vi "4461 Sim - Noise.vi"(4 "Noise Cluster":T1={"1/f vs. Uniform "=1.0, "DC Drift Fraction"=0.0, "DC Drift Freq"=0.19999999999999996, "DC Offset"=0.0, "60Hz Amplitude"=0.005, "Gauss/Unif %"=0.5, "Sig Amp"=1.0, "Noise Amp"=0.005} {"Noise Amp" format="%.1p"; "Sig Amp" format="%.2p"; "Gauss/Unif %" min=0.0 max=1.0 step=0.05 format="%.2f"; "60Hz Amplitude" min=0.0 max=10.0 step=0.05 format="%.2p"; "DC Offset" min=-1.0 max=1.0 step=0.01 format="%.2f"; "DC Drift Freq" min=0.0 max=5.0 step=0.05 format="%.2f"; "DC Drift Fraction" format="%.2f"; "1/f vs. Uniform" min=0.0 max=50.0 step=0.5 format="%.1p"}, 5 "data":waveform(dbl)[](array[waveform]), 6 "sampling info":cluster{"Fs":dbl, "#s":dbl}={"Fs"=204800.0, "#s"=20480.0}) -> (0 "Data":waveform(dbl)[](array[waveform]))   [LabVIEW 2016]
uses:
  <vilib>/Analysis/2dsp.llb/Real FFT.vi
  <vilib>/Analysis/2dsp.llb/Inverse Real FFT.vi
  <vilib>/Analysis/2dsp.llb/Decimate (single shot).vi
  <vilib>/Analysis/2dsp.llb/Decimate (single shot, DBL).vi
  <vilib>/Analysis/3filter.llb/Butterworth Filter (DBL).vi
  <vilib>/Utility/error.llb/Error Cluster From Error Code.vi
  <vilib>/measure/NI_MABase.lvlib
  <vilib>/Analysis/NI_AALPro.lvlib
  <vilib>/Analysis/NI_AALBase.lvlib
panel:
  out "Waveform Graph 2":waveform(dbl)[](graph)
  out "Waveform Graph":waveform(dbl)[](graph)
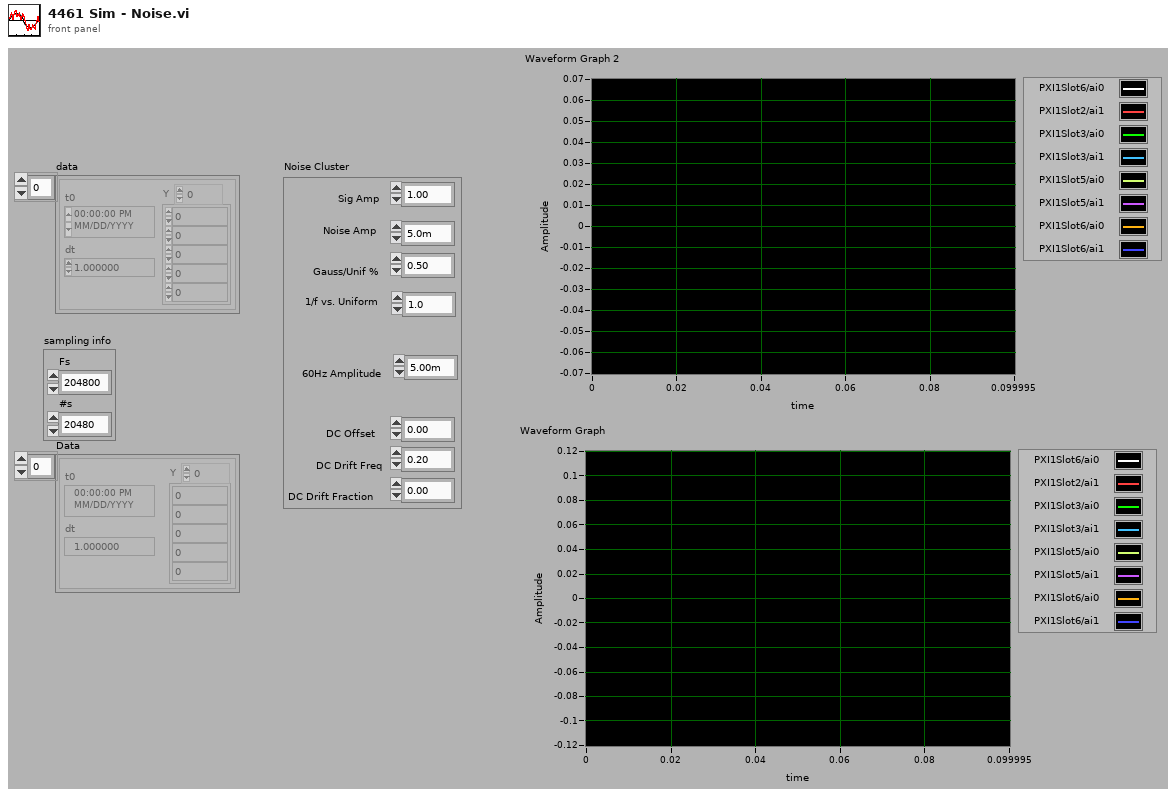
[diagram p1: front panel]
types:
  T1 = cluster{"1/f vs. Uniform ":dbl, "DC Drift Fraction":dbl, "DC Drift Freq":dbl, "DC Offset":dbl, "60Hz Amplitude":dbl, "Gauss/Unif %":dbl, "Sig Amp":dbl, "Noise Amp":dbl}
  T2 = enum32{"Lowpass", "Highpass", "Bandpass", "Bandstop"}
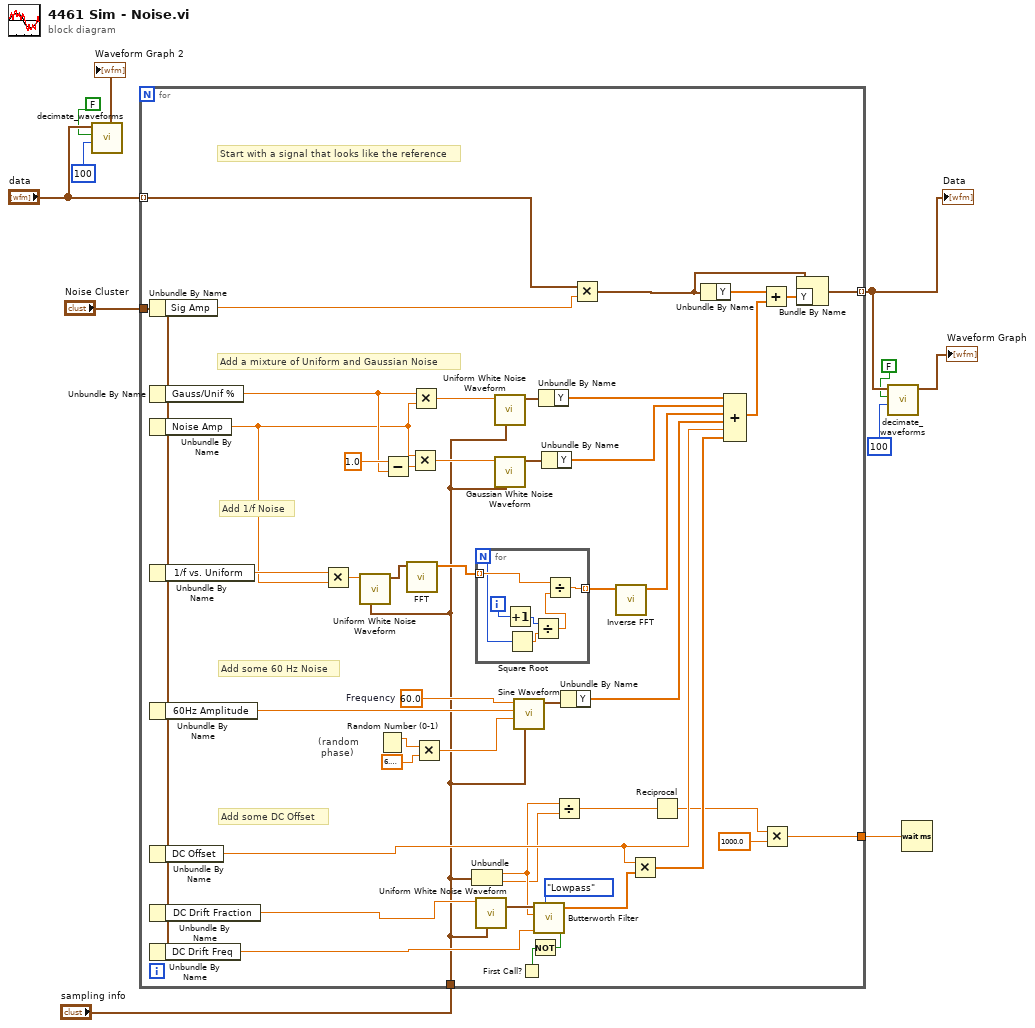
[diagram p0: block diagram]
diagram:
  n1 = call "decimate_waveforms.vi"("Input Signal"="data", "averaging"=FALSE, "decimating factor"=100) -> ("Decimated Waveforms"=→"Waveform Graph 2":waveform(dbl)[])  [unwired: 6 in, 1 out]
  n2 = for {
    tunnel: "Noise Cluster" -> [w27]
    tunnel: "sampling info" -> [w24]
    tunnel: "data" -> [w22] mode=indexing
    tunnel: [w18] -> w9 mode=indexing
    tunnel: [w12] -> w5
    w52 = 60.0  # Frequency
    # "Start with a signal that looks like the reference"
    # "Add 1/f Noise"
    # "(random\n phase)"
    # "Add some DC Offset"
    # "Add some 60 Hz Noise"
    # "Add a mixture of Uniform and Gaussian Noise"
    n3 = Unbundle By Name(w27) -> ("Sig Amp"=w23:dbl)
    n4 = Unbundle By Name(w27) -> ("Gauss/Unif %"=w32:dbl)
    n5 = Unbundle By Name(w27) -> ("Noise Amp"=w30:dbl)
    n6 = Unbundle By Name(w27) -> ("1/f vs. Uniform"=w31:dbl)
    n7 = Unbundle By Name(w27) -> ("60Hz Amplitude"=w29:dbl)
    n8 = Unbundle By Name(w27) -> ("DC Offset"=w28:dbl)
    n9 = Unbundle By Name(w27) -> ("DC Drift Fraction"=w25:dbl)
    n10 = Unbundle By Name(w27) -> ("DC Drift Freq"=w26:dbl)
    n11 = Multiply(x=w31, y=w30) -> (x*y=w40:dbl)
    n12 = call <vilib>:"Uniform White Noise Waveform.vi"("sampling info"=w24, "amplitude"=w40) -> ("signal out"=w39:waveform(dbl))  [unwired: 8 in, 1 out]
    n13 = Random Number (0-1)() -> (number: 0 to 1=w50:dbl)
    n14 = Subtract(x=1.0, y=w32) -> (x-y=w54:dbl)
    n15 = call-poly <vilib>:"FFT.vi"("X"=w39) -> ("FFT {X}"=w42:cdb[])  [unwired: 9 in, 1 out]
    n16 = Multiply(x=w30, y=w54) -> (x*y=w56:dbl)
    n17 = Multiply(x=w32, y=w30) -> (x*y=w55:dbl)
    n18 = Multiply(x=w50, y=6.283185307179586) -> (x*y=w49:dbl)
    n19 = Unbundle(w24) -> ("Fs"=w15:dbl, "#s"=w14:dbl)
    n20 = for {
      N -> [w62]
      tunnel: [w65] -> w41 mode=indexing
      tunnel: w42 -> [w64] mode=indexing
      i -> [w63]
      n21 = Increment(x=w63) -> (x+1=w60:i32)
      n22 = Square Root(x=w62) -> (sqrt(x)=w61:dbl)
      n23 = Divide(x=w60, y=w61) -> (x/y=w59:dbl)
      n24 = Divide(x=w64, y=w59) -> (x/y=w65:cdb)
    }
    n25 = call <vilib>:"Uniform White Noise Waveform.vi"("sampling info"=w24, "amplitude"=w25) -> ("signal out"=w47:waveform(dbl))  [unwired: 8 in, 1 out]
    n26 = call <vilib>:"Uniform White Noise Waveform.vi"("sampling info"=w24, "amplitude"=w55) -> ("signal out"=w57:waveform(dbl))  [unwired: 8 in, 1 out]
    n27 = call <vilib>:"Gaussian White Noise Waveform.vi"("sampling info"=w24, "standard deviation"=w56) -> ("signal out"=w58:waveform(dbl))  [unwired: 8 in, 1 out]
    n28 = call <vilib>:"Sine Waveform.vi"("sampling info"=w24, "phase"=w49, "amplitude"=w29, "frequency"=w52) -> ("signal out"=w48:waveform(dbl))  [unwired: 6 in, 1 out]
    n29 = First Call?() -> (First Call?: T/F=w33:bool)
    n30 = Not(x=w33) -> (.not. x?=w45:bool)
    n31 = call-poly <vilib>:"Butterworth Filter.vi"("init/cont (init:F)"=w45, "filter type"=T2."Lowpass", "low cutoff freq: fl"=w26, "sampling freq: fs"=w15, "X"=w47) -> ("Filtered X"=w44:dbl[])  [unwired: 3 in, 1 out]
    n32 = Unbundle By Name(w57) -> ("Y"=w43:dbl[])
    n33 = Unbundle By Name(w58) -> ("Y"=w34:dbl[])
    n34 = Divide(x=w15, y=w14) -> (x/y=w13:dbl)
    n35 = Unbundle By Name(w48) -> ("Y"=w38:dbl[])
    n36 = Multiply(x=w22, y=w23) -> (x*y=w19:waveform(dbl))
    n37 = call-poly <vilib>:"Inverse FFT.vi"("FFT {X}"=w41) -> ("X"=w37:dbl[])  [unwired: 9 in, 1 out]
    n38 = Multiply(x=w28, y=w44) -> (x*y=w36:dbl[])
    n39 = Reciprocal(x=w13) -> (1/x=w16:dbl)
    n40 = Unbundle By Name(w19) -> ("Y"=w21:dbl[])
    n41 = Compound Arithmetic op=ADD(w43, w34, w37, w38, w28, w36) -> (w35:dbl[])
    n42 = Add(x=w21, y=w35) -> (x+y=w20:dbl[])
    n43 = Multiply(x=w16, y=1000.0) -> (x*y=w12:dbl)
    n44 = Bundle By Name(cluster=w19, "Y"=w20) -> (w18:waveform(dbl))
  }
  "Data" <- w9
  n45 = call "decimate_waveforms.vi"("Input Signal"=w9, "averaging"=FALSE, "decimating factor"=100) -> ("Decimated Waveforms"=→"Waveform Graph":waveform(dbl)[])  [unwired: 6 in, 1 out]
  n46 = Wait (ms)(milliseconds to wait=w5) -> ()  [unwired: 1 out]
